vi "VectorNav parse QMA broken.vi"(11 "input data":u8) -> ()   [LabVIEW 2010]
uses:
  VectorNav parse QMA state typedef.vi
panel:
  out "count":u8
  out "Array":u8[](array[numeric])
  out "Boolean":bool
  out "data array length":u8
  out "data array":u8[](array[numeric])
  # "change i can believe in!"
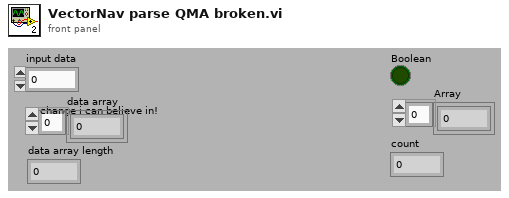
[diagram p1: front panel]
types:
  T1 = typedef "VectorNav parse QMA state typedef.vi" = enum16{"wait for $", "confirm command", "q[0] of quaternion", "q[1] of quaternion", "q[2] of quaternion", "q[3] of quaternion (scalar term)", "X-Axis Magnetic", "Y-Axis Magnetic", "Z-Axis Magnetic", "X-Axis Acceleration", "Y-Axis-Acceleration", "Z-Axis-Acceleration", "Checksum"}
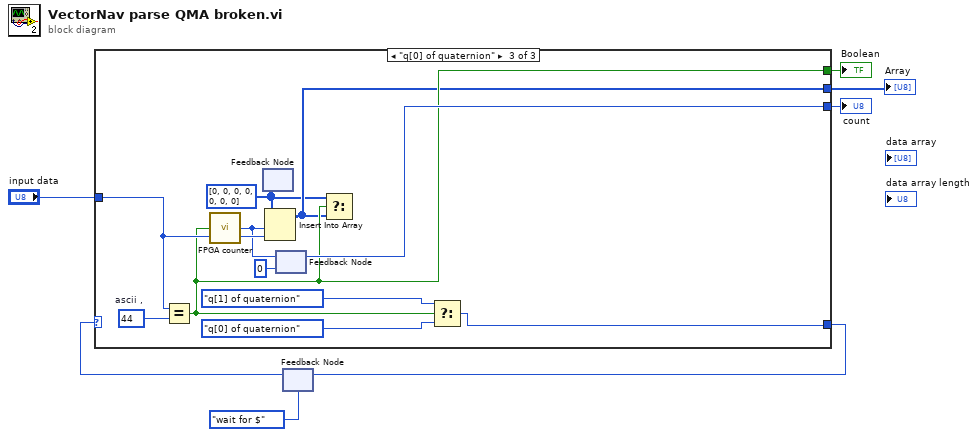
[diagram p0: block diagram]
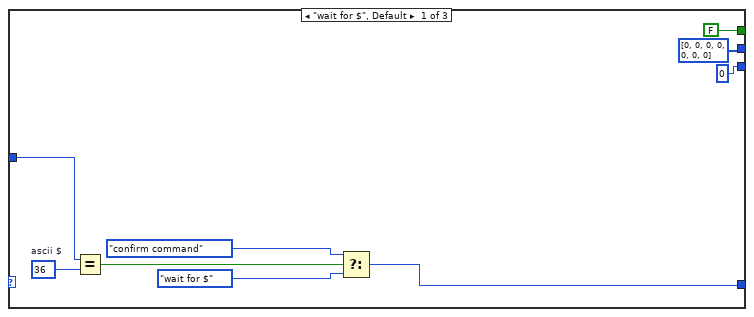
[diagram p2: hidden frame]
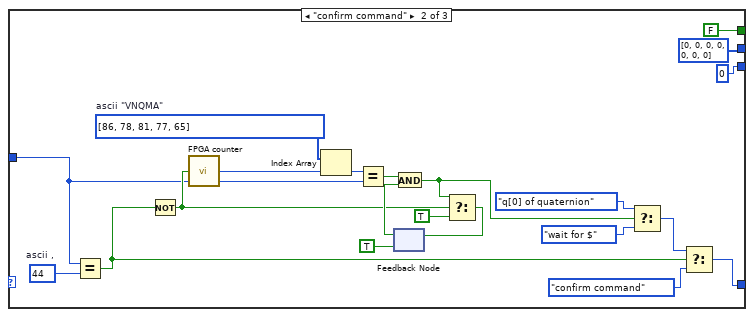
[diagram p3: hidden frame]
diagram:
  n1 = feedback #1(VectorNav_parse_QMA_state_typedef.vi."wait for $" ("Enum")) -> (w6:T1)
  n2 = case shown="\"q[0] of quaternion\"" w6 {
    tunnel: "input data" -> [w16 w24 w44]
    tunnel: [w11 w32 w45] -> w4
    tunnel: [FALSE FALSE w41] -> w3
    tunnel: [u8[] [0, 0, 0, 0, 0, 0, 0] ("Array") u8[] [0, 0, 0, 0, 0, 0, 0] ("Array") w39] -> w2
    tunnel: [u8 0 ("count") u8 0 ("count") w42] -> w1
    frame "wait for $", Default {
      w15 = u8 36  # ascii $
      n3 = Equal?(x=w16, y=w15) -> (x = y?=w14:bool)
      n4 = Select(t=VectorNav_parse_QMA_state_typedef.vi."confirm command" ("Enum"), s=w14, f=VectorNav_parse_QMA_state_typedef.vi."wait for $" ("Enum")) -> (s? t:f=w11:T1)
    }
    frame "confirm command" {
      w22 = u8[] [86, 78, 81, 77, 65]  # ascii "VNQMA"
      w37 = u8 44  # ascii ,
      n5 = Equal?(x=w24, y=w37) -> (x = y?=w23:bool)
      n6 = Not(x=w23) -> (.not. x?=w28:bool)
      n7 = call "FPGA counter.vi"("no reset?"=w28) -> ("count"=w25:u8)
      n8 = Index Array(array=w22, index=w25) -> (element=w26:u8)
      n9 = Equal?(x=w26, y=w24) -> (x = y?=w27:bool)
      n10 = feedback #2(TRUE ("f")) -> (w30:bool)
      n11 = And(x=w27, y=w30) -> (x .and. y?=w20:bool)
      n12 = Select(t=w20, s=w28, f=TRUE) -> (s? t:f=w21:bool)
      n13 = feedback-in #2(w21) -> ()
      n14 = Select(t=VectorNav_parse_QMA_state_typedef.vi."q[0] of quaternion" ("Enum"), s=w20, f=VectorNav_parse_QMA_state_typedef.vi."wait for $" ("Enum")) -> (s? t:f=w33:T1)
      n15 = Select(t=w33, s=w23, f=VectorNav_parse_QMA_state_typedef.vi."confirm command" ("Enum")) -> (s? t:f=w32:T1)
    }
    frame "q[0] of quaternion" {
      w38 = u8[] [0, 0, 0, 0, 0, 0, 0]
      w48 = u8 44  # ascii ,
      n16 = Equal?(x=w44, y=w48) -> (x = y?=w41:bool)
      n17 = call "FPGA counter.vi"("no reset?"=w41) -> ("count"=w43:u8)
      n18 = feedback-in #3(w38) -> ()
      n19 = feedback #3(w38, w38) -> ()
      n20 = Insert Into Array(array=w38, index=w43, new element=w44) -> (w39:u8[])
      n21 = feedback-in #4(w43) -> ()
      n22 = feedback #4(u8 0 ("count")) -> (w42:u8)
      n23 = Select(t=w38, s=w41, f=w39) -> ()  [unwired: 1 out]
      n24 = Select(t=VectorNav_parse_QMA_state_typedef.vi."q[1] of quaternion" ("Enum"), s=w41, f=VectorNav_parse_QMA_state_typedef.vi."q[0] of quaternion" ("Enum")) -> (s? t:f=w45:T1)
    }
  }
  "Boolean" <- w3
  "Array" <- w2
  "count" <- w1
  n25 = feedback-in #1(w4) -> ()
